vi "7HP_Pressures_to UVW.vi"(3 "Probe Number":i32) -> (1 "UVW chs":i32[](array[numeric]))   [LabVIEW 2021]
uses:
  Controls/Post_Process.ctl
  Controls/Setup.ctl
  Data plotting/MATLAB/MATLAB_Mode.ctl
  Sub_vis/Upload Data.ctl
  <vilib>/Analysis/baseanly.llb/Mean (DBL).vi
  Globals/Meas_global.vi
  Analysis/7 Hole Probe pressures to UVW/7HP_Global.vi
  Globals/Constants_global.vi
  <vilib>/Analysis/NI_AALBase.lvlib
panel:
  out "Uncorrected UVW":sgl[](array[numeric]) format="%.4f"
  out "Time to Run (s)":dbl format="%.1f"
  out "Modified Calib filename":string
  out "UVW Data?":bool
  out "RD UVW file":path
  out "RD Pressure file":path
  out "Size":i32
  out "Calib last mod":timestamp
  in  "Plot Traces":bool
  out "Array":T1(array[cluster])
  out "UVW Filepath":path
  out "UVW Sampling Rate Hz":sgl
  out "Serial number":u32
  out "Calib File":path
  out "Relative yaw (deg)":sgl
  out "Relative pitch (deg)":sgl
  out "Relative roll (deg)":sgl
  out "Calib. pitch (deg)":sgl
  out "Calib. roll (deg)":sgl
  out "Pitch (deg)":sgl
  out "Roll (deg)":sgl
  in  "Desired Freq Hz":sgl=50.0
  out "Averaging samples":i32=5
  out "Current Case":string
  out "7 Hole Probe chs":string[](array[string])
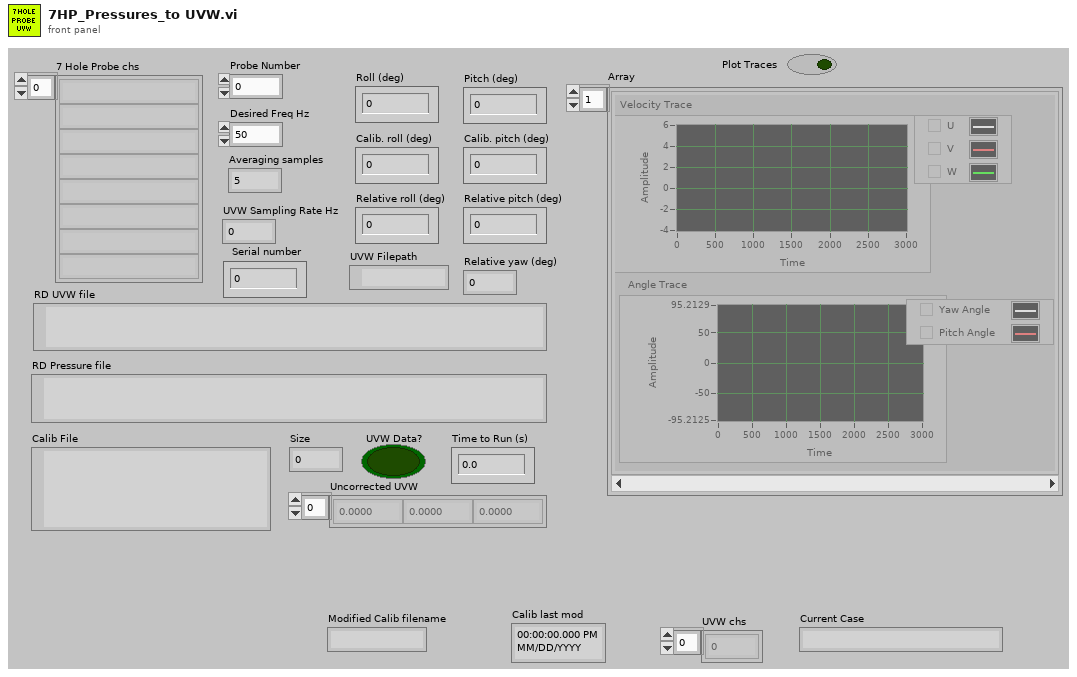
[diagram p1: front panel]
types:
  T1 = cluster{"Angle Trace":dbl[][], "Velocity Trace":sgl[][]}[]
  T2 = typedef "Post_Process.ctl" = enum16{"Take New Data", "Post Process Raw Data File"}
  T3 = typedef "Analysis_info_cluster.ctl" = cluster{"Colour":u32, "Inst type":T4, "Inst name":string, "Symbol":string, "Code name":string, "Extra Info":string, "Inst Array":T5, "Extra Titles":string[], "Extra Values":string[], "U":dbl, "u^2":dbl, "u^3":dbl, "u^4":dbl, "Skew_u":dbl, "Kurt_u":dbl, "Sd Error in Mean":dbl, "% u'/U":dbl, "X":dbl, "Y":dbl, "Z":dbl, "Timescale integral Estimate":dbl, "Sd Error in Variance":dbl, "Calib File":path, "Calib Constants":dbl[], "Output Position":bool, "Stats":enum16{"None", "Basic", "Full"}, "Av Sampling Rate":dbl, "Av No of Samples":dbl, "Total Meas Time (s)":dbl, "ADAM Ch Name":string, "Max value":dbl, "Min value":dbl, "Req Sample Rate Hz":dbl, "Sync Delay Time (s)":dbl, "Ch No":i16, "Device":string, "Use Latest Calib":bool, "Port":string, "Metadata Ch Names":string[], "Metadata Ch Values":string[], "Label":string}
  T4 = typedef "Inst_type.ctl" = enum16{"Raw voltage", "Raw with zero offsetting", "Propeller anemometer", "Pressure Transducer", "Pitot-static tube", "Hot wire", "Cross wire 1", "Cross wire 2", "Generic Linear", "Generic Polynomial", "Generic BackPoly", "Fast FID", "Thermocouple", "Cold wire", "Pulsed Wire", "LDA Vel", "LDA Tran time", "LDA Arr time", "Microphone"}
  T5 = typedef "Instrument_Array.ctl" = enum16{"PWA", "LDA", "Analogue"}
  T6 = typedef "Time_Trace_Cluster.ctl" = cluster{"Weighting":dbl[], "Voltage":dbl[], "Eng Values":dbl[]}
  T7 = typedef "Setup.ctl" = enum16{"Run Program", "Show Setup", "Save Current Setup", "Setup Front Panel"}
  T8 = enum16{"Save no data", "Save data in new files", "Save data in existing files"}
  T9 = typedef "MATLAB_Mode.ctl" = enum16{"1D Plotter", "2D Plotter", "LP Plotter", "7HP UVW"}
  T10 = typedef "Upload Data.ctl" = enum16{"Voltage Array", "Time Trace Cluster"}
  T11 = cluster{"Angle Trace":dbl[][], "Velocity Trace":sgl[][]}
  T12 = cluster{"Pressure Ch Names":string[], "Pressure Index":i32[], "Metadata Index":i32[], "Port":string}[]
  T13 = cluster{"Pressure Ch Names":string[], "Pressure Index":i32[], "Metadata Index":i32[], "Port":string}
  T14 = typedef "LVDateTimeRec.ctl" = cluster{"fractional second":dbl, "second":i32, "minute":i32, "hour":i32, "day of month":i32, "month":i32, "year":i32, "day of week":i32, "day of year":i32, "DST":i32}
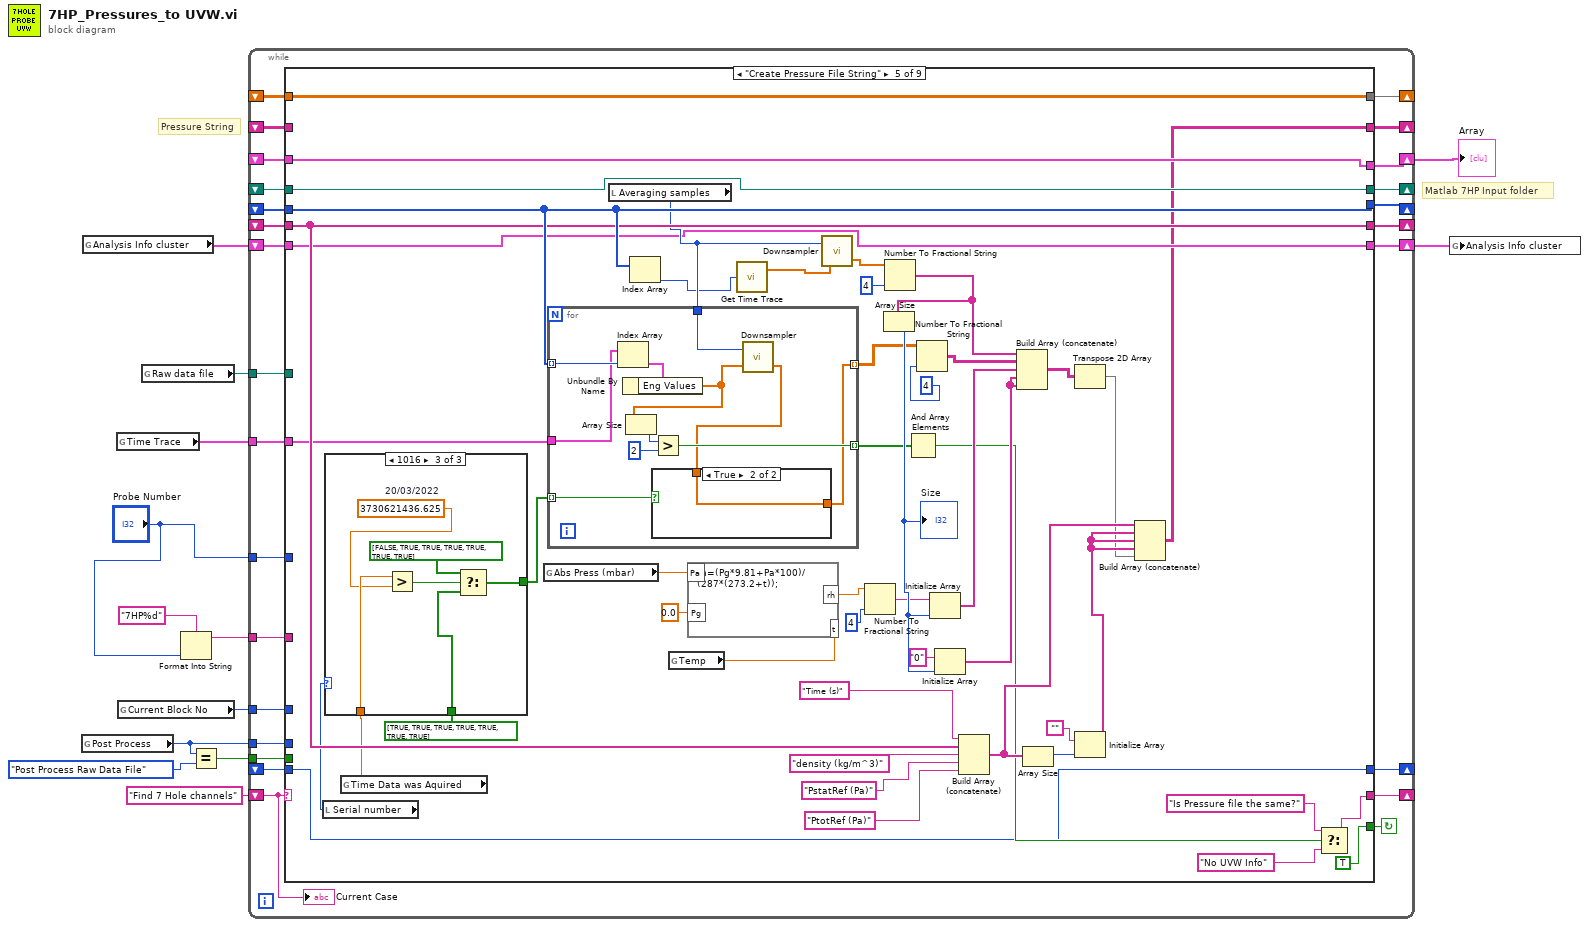
[diagram p0: block diagram]
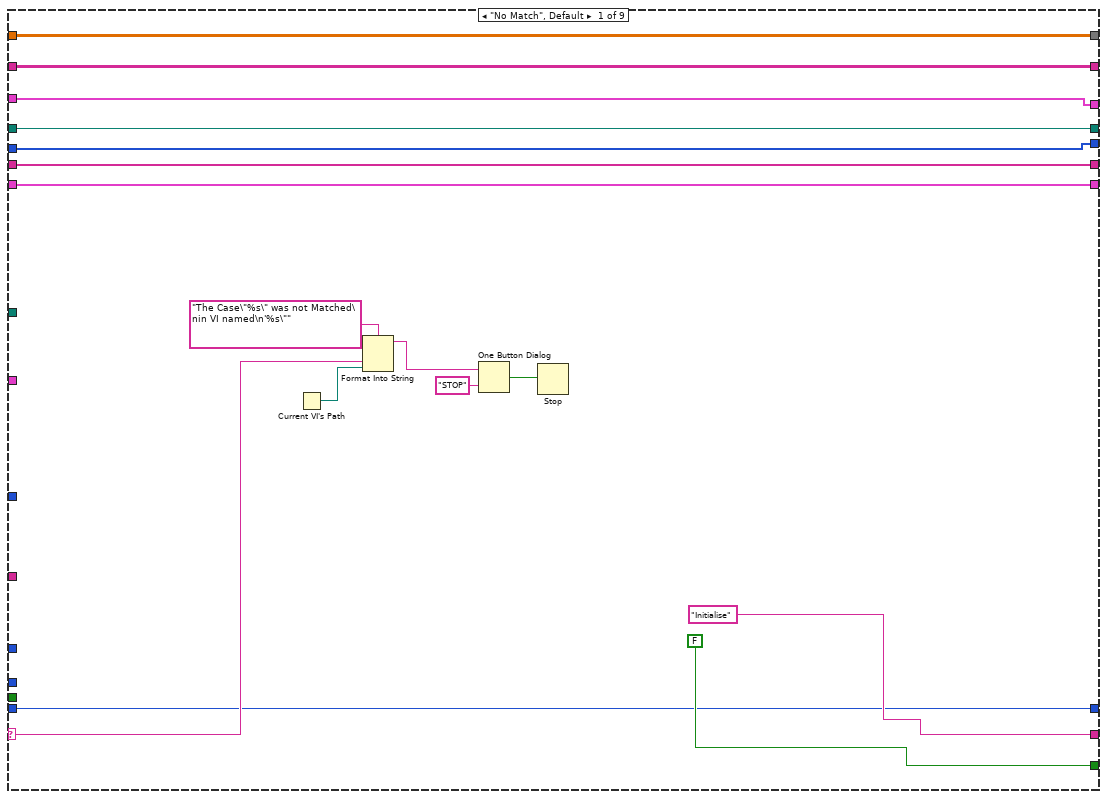
[diagram p2: hidden frame]
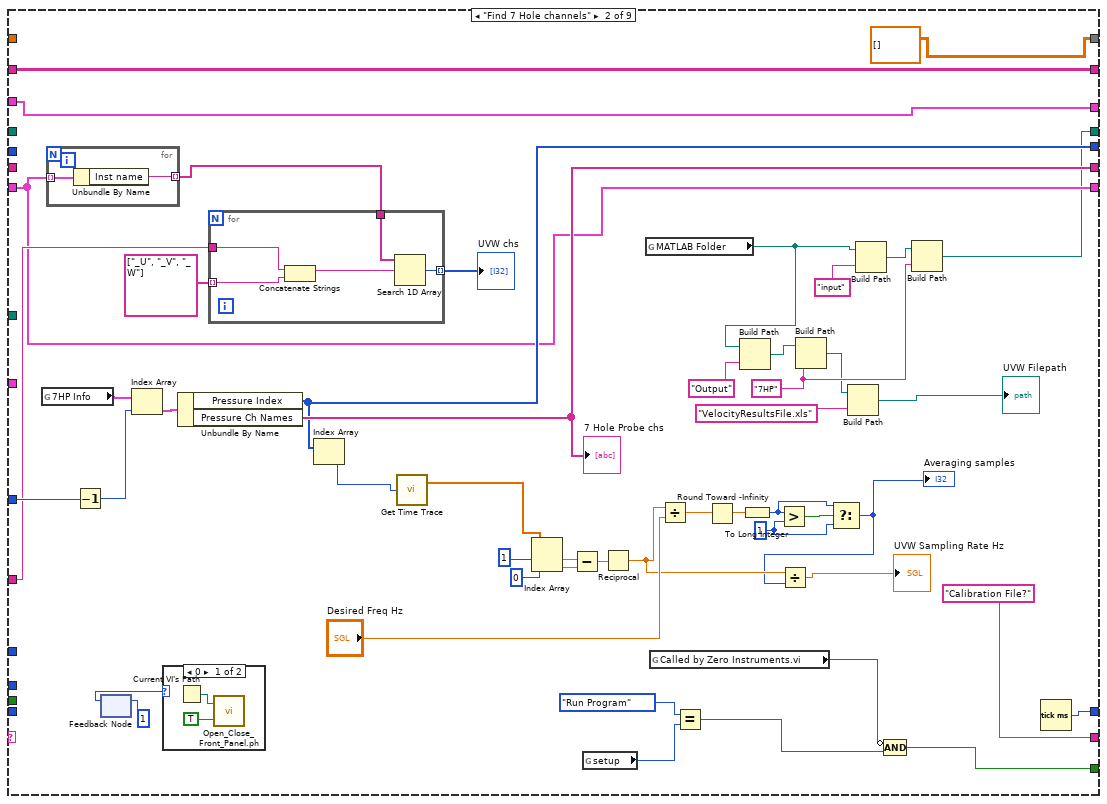
[diagram p3: hidden frame]
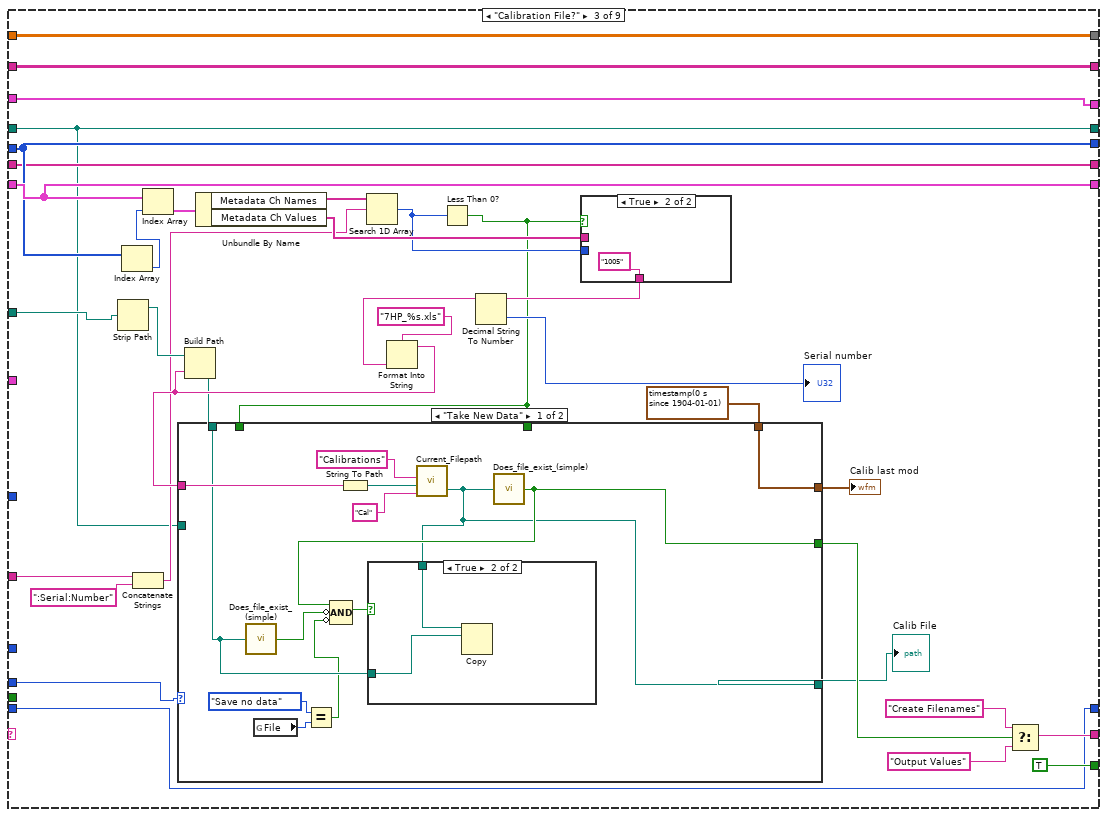
[diagram p5: hidden frame]
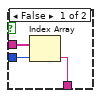
[diagram p6: hidden frame]
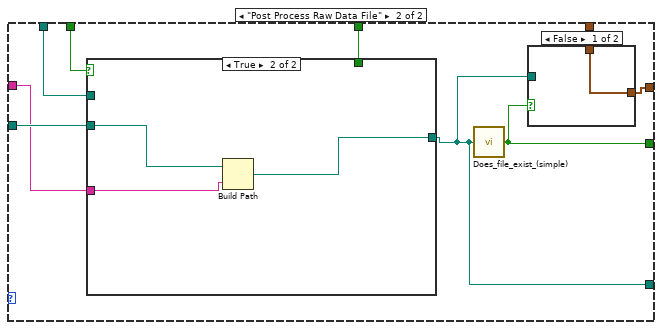
[diagram p8: hidden frame]
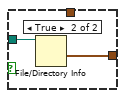
[diagram p9: hidden frame]
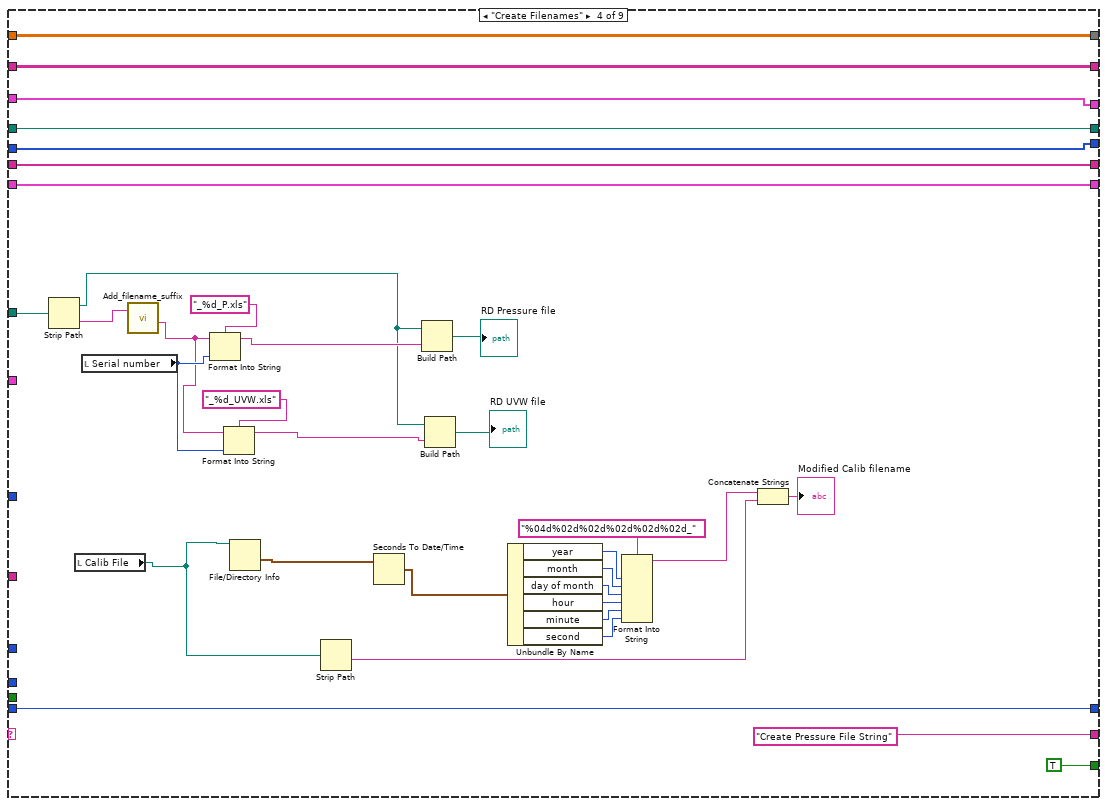
[diagram p11: hidden frame]
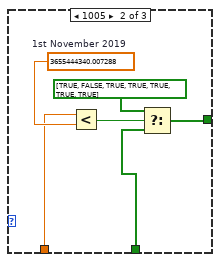
[diagram p13: hidden frame]
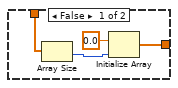
[diagram p14: hidden frame]
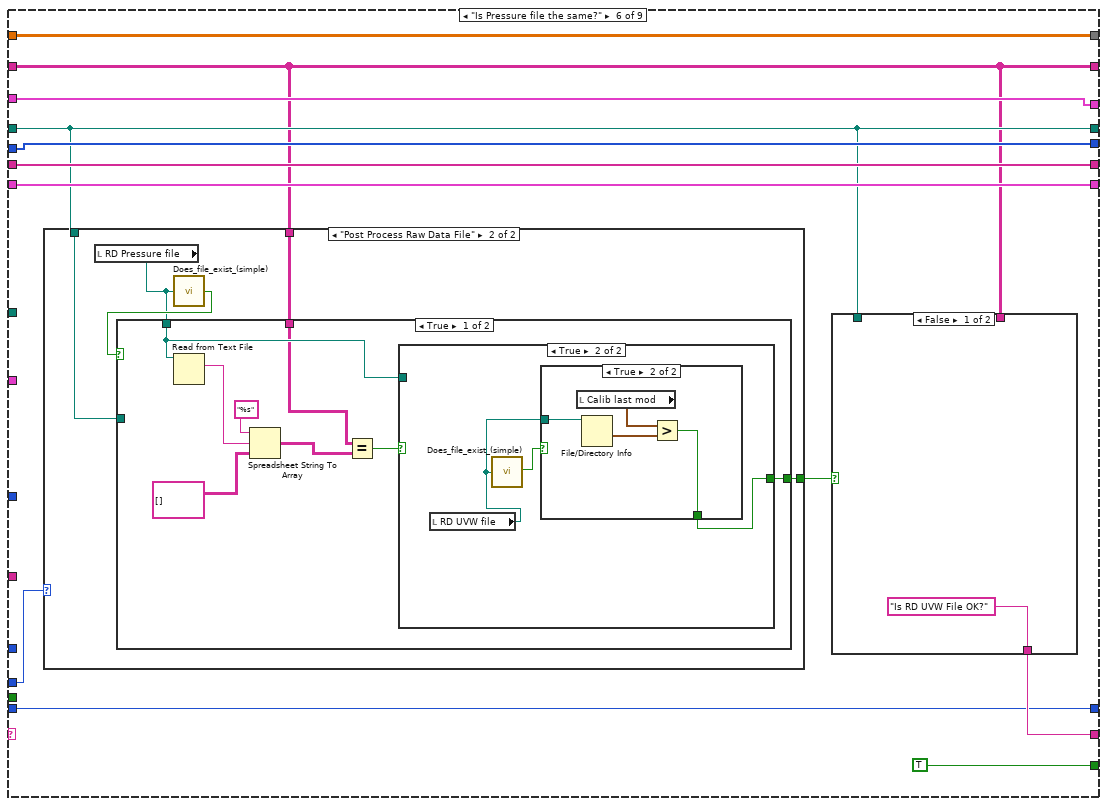
[diagram p15: hidden frame]
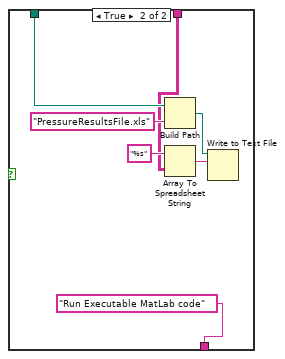
[diagram p16: hidden frame]
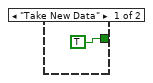
[diagram p17: hidden frame]
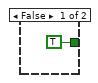
[diagram p18: hidden frame]
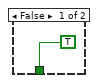
[diagram p19: hidden frame]
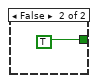
[diagram p20: hidden frame]
diagram:
  # "Matlab 7HP Input folder"
  # "Pressure String"
  n1 = global read "Meas_global.vi" "Post Process"() -> (w4:T2)
  n2 = global read "Meas_global.vi" "Analysis Info cluster"() -> (w3:T3[])
  n3 = global read "Meas_global.vi" "Time Trace"() -> (w11:T6[])
  n4 = global read "Meas_global.vi" "Current Block No"() -> (w10:i32)
  n5 = global read "Meas_global.vi" "Raw data file"() -> (w12:path)
  n6 = Format Into String(format string="7HP%d", "Probe Number") -> (resulting string=w8:string)  [unwired: 2 in, 1 out]
  n7 = Equal?(x=w4, y=Post_Process."Post Process Raw Data File" ("Post Process")) -> (x = y?=w5:bool)
  n8 = while {
    shift-left: "Find 7 Hole channels" -> [w28]
    shift-right: [w29] -> _
    tunnel: w12 -> [w38]
    shift-right: [w37] -> _
    shift-left: _ -> [w36]
    shift-right: [w35] -> _
    shift-left: _ -> [w34]
    shift-right: [w33] -> _
    shift-left: _ -> [w32]
    tunnel: w11 -> [w31]
    tunnel: w10 -> [w30]
    tunnel: "Probe Number" -> [w27]
    tunnel: w8 -> [w26]
    tunnel: w5 -> [w25]
    tunnel: w4 -> [w24]
    shift-right: [w22] -> w2
    shift-left: w3 -> [w23]
    shift-right: [w20] -> w1
    shift-left: _ -> [w21]
    shift-right: [w19] -> _
    shift-left: _ -> [w18]
    shift-right: [w17] -> _
    shift-left: _ -> [w16]
    shift-right: [w15] -> _
    shift-left: _ -> [w14]
    stop <- w39 continue-if-true
    n9 = case shown="\"Create Pressure File String\"" w28 {
      selector: w28 -> [w45 _ _ _ _ _ _ _ _]
      tunnel: [FALSE w71 TRUE TRUE TRUE TRUE TRUE TRUE FALSE] -> w39
      tunnel: ["Initialise" "Calibration File?" ("t") w131 "Create Pressure File String" ("t") w227 w294 w344 "Output Values" ("t") w445] -> w29
      tunnel: w38 -> [_ _ w136 w204 _ _ _ _ w442]
      tunnel: [w48 w93 w139 w213 w262 w303 w356 w381 w436] -> w37
      tunnel: w36 -> [w48 _ w139 w213 w262 w303 w356 w381 w443]
      tunnel: [w47 w100 w138 w212 w242 w304 w358 w382 w447] -> w35
      tunnel: w34 -> [w47 _ w138 w212 w242 w304 w358 w382 w447]
      tunnel: [w46 w80 w122 w214 w232 w296 w339 w377 w435] -> w33
      tunnel: w32 -> [w46 _ w122 w214 w232 w296 w339 w377 w434]
      tunnel: w31 -> [_ _ _ _ w236 _ _ _ w444]
      tunnel: w30 -> [_ _ _ _ _ _ _ _ _]
      tunnel: w27 -> [_ w94 _ _ _ _ _ _ w441]
      tunnel: w26 -> [_ w92 w128 _ _ _ _ _ w440]
      tunnel: w25 -> [_ _ _ _ _ _ _ _ _]
      tunnel: w24 -> [_ _ w141 _ _ w301 _ w379 _]
      tunnel: w23 -> [w44 w87 w140 w211 w233 w302 w355 w380 w438]
      tunnel: [w44 w87 w140 w211 w233 w302 w355 w380 w439] -> w22
      tunnel: w21 -> [w43 w85 w120 w215 w231 w299 w354 w376 w433]
      tunnel: [w43 w85 w120 w215 w231 w299 w354 w376 w432] -> w20
      tunnel: [w42 w84 w117 w209 w223 w295 w338 w375 w431] -> w19
      tunnel: w18 -> [w42 w84 w117 w209 _ w295 w338 w375 w431]
      tunnel: [w41 sgl[][] [] w116 w199 w224 w298 w341 w373 w430] -> w17
      tunnel: w16 -> [w41 _ w116 w199 w224 w298 w340 w372 w430]
      tunnel: [w40 w75 w115 w182 w222 w293 w337 w369 w429] -> w15
      tunnel: w14 -> [w40 _ w115 w182 w222 w293 w337 w369 w429]
      frame "No Match", Default {
        n10 = Current VI's Path() -> (path=w50:path)
        n11 = Format Into String(format string="The Case\"%s\" was not Matched\nin VI named\n'%s\"" ("Format String"), w45, w50) -> (resulting string=w53:string)  [unwired: 2 in, 1 out]
        n12 = One Button Dialog(message=w53, button name ("OK")="STOP") -> (true=w51:bool)
        n13 = Stop(stop? (T)=w51) -> ()
      }
      frame "Find 7 Hole channels" {
        w59 = 1 ("y")
        w77 = "7HP" ("name or relative path")
        n14 = global read "7HP_Global.vi" "7HP Info"() -> (w86:T12)
        n15 = for {
          tunnel: w87 -> [w108] mode=indexing
          tunnel: [w107] -> w96 mode=indexing
          n16 = Unbundle By Name(w108) -> ("Inst name"=w107:string)
        }
        n17 = Decrement(x=w94) -> (x-1=w98:i32)
        n18 = feedback-in #1(1) -> ()
        n19 = feedback #1() -> (w90:i32)  [unwired: 1 in]
        n20 = Index Array(array=w86, index=w98) -> (element=w101:T13)
        n21 = case shown="0" w90 {
          frame 0 {
            n22 = Current VI's Path() -> (path=w105:path)
            n23 = call "Open_Close_Front_Panel.ph.vi"("openWindow (T)"=TRUE ("Front Panel Window:Open"), "VI path"=w105) -> ()  [unwired: 1 in, 1 out]
          }
          frame Default {
          }
        }
        n24 = Unbundle By Name(w101) -> ("Pressure Index"=w93:i32[], "Pressure Ch Names"=w100:string[])
        "7 Hole Probe chs" <- w100
        n25 = for {
          tunnel: string[] ["_U", "_V", "_W"] ("appended array") -> [w113] mode=indexing
          tunnel: w96 -> [w112]
          tunnel: [w110] -> w95 mode=indexing
          tunnel: w92 -> [w109]
          n26 = Concatenate Strings(w109, w113) -> (w111:string)
          n27 = Search 1D Array(1D array=w112, element=w111) -> (index of element=w110:i32)  [unwired: 1 in]
        }
        "UVW chs" <- w95
        n28 = Index Array(array=w93) -> (element=w57:i32)  [unwired: 1 in]
        n29 = call "Get Time Trace.vi"("Channel Index"=w57) -> ("Time (s)"=w56:dbl[])  [unwired: 1 out]
        n30 = Index Array(array=w56, index #1=1 ("index"), index #2=0 ("index")) -> (element #1=w66:dbl, element #2=w67:dbl)
        n31 = Subtract(x=w66, y=w67) -> (x-y=w65:dbl)
        n32 = global read "Meas_global.vi" "setup"() -> (w103:T7)
        n33 = Reciprocal(x=w65) -> (1/x=w64:dbl)
        n34 = global read "Constants_global.vi" "MATLAB Folder"() -> (w74:path)
        n35 = global read "Meas_global.vi" "Called by Zero Instruments.vi"() -> (w73:bool)
        n36 = Divide(x=w64, y="Desired Freq Hz") -> (x/y=w99:dbl)
        n37 = Equal?(x=Setup."Run Program" ("setup"), y=w103) -> (x = y?=w72:bool)
        n38 = Round Toward -Infinity(1:w99) -> (0:w63:dbl)
        n39 = Build Path(base path=w74, name or relative path="Output") -> (appended path=w79:path)
        n40 = To Long Integer(number=w63) -> (32bit integer=w60:i32)
        n41 = Greater?(x=w60, y=w59) -> (0:w61:bool)
        n42 = Build Path(base path=w79, name or relative path=w77) -> (appended path=w76:path)
        n43 = Select(t=w60, s=w61, f=w59) -> (s? t:f=w58:i32)
        "Averaging samples" <- w58
        n44 = Divide(x=w64, y=w58) -> (x/y=→"UVW Sampling Rate Hz":dbl)
        n45 = Build Path(base path=w76, name or relative path="VelocityResultsFile.xls") -> (appended path=→"UVW Filepath":path)
        n46 = Build Path(base path=w74, name or relative path="input") -> (appended path=w81:path)
        n47 = Compound Arithmetic op=AND(invert w73, w72) -> (w71:bool)
        n48 = Build Path(base path=w81, name or relative path=w77) -> (appended path=w80:path)
        n49 = Tick Count (ms)() -> (millisecond timer value=w75:u32)
      }
      frame "Calibration File?" {
        n50 = Strip Path(path=w136) -> (stripped path=w137:path)  [unwired: 1 out]
        n51 = Index Array(array=w139) -> (element=w146:i32)  [unwired: 1 in]
        n52 = Concatenate Strings(w128, ":Serial:Number") -> (w127:string)
        n53 = Index Array(array=w140, index=w146) -> (element=w145:T3)
        n54 = Unbundle By Name(w145) -> ("Metadata Ch Names"=w144:string[], "Metadata Ch Values"=w143:string[])
        n55 = Search 1D Array(1D array=w144, element=w127) -> (index of element=w125:i32)  [unwired: 1 in]
        n56 = Less Than 0?(x=w125) -> (x < 0?=w123:bool)
        n57 = case shown="True" w123 {
          tunnel: w143 -> [w149 _]
          tunnel: w125 -> [w148 _]
          tunnel: [w147 "1005" ("String")] -> w124
          frame False {
            n58 = Index Array(array=w149, index=w148) -> (element=w147:string)
          }
          frame True {
          }
        }
        n59 = Format Into String(format string="7HP_%s.xls", w124) -> (resulting string=w135:string)  [unwired: 2 in, 1 out]
        n60 = Build Path(base path=w137, name or relative path=w135) -> (appended path=w134:path)
        n61 = case shown="\"Take New Data\"" w141 {
          tunnel: w135 -> [w160 w170]
          tunnel: [w159 w168] -> w132
          tunnel: w134 -> [w156 w173]
          tunnel: w123 -> [_ w174]
          tunnel: w123 -> [_ w172]
          tunnel: w122 -> [_ w171]
          tunnel: [w155 w169] -> w121
          tunnel: timestamp(0 s since 1904-01-01) ("last mod") -> [w151 w166]
          tunnel: [w151 w167] -> w118
          frame "Take New Data" {
            n62 = call "Does_file_exist_(simple).vi"("Pathname"=w156) -> ("exists?"=w158:bool)
            n63 = global read "Meas_global.vi" "File"() -> (w154:T8)
            n64 = Equal?(x=T8."Save no data" ("File"), y=w154) -> (x = y?=w152:bool)
            n65 = String To Path(string=w160) -> (path=w163:path)
            n66 = call "Current_Filepath.vi"("Short_Name"="Cal" ("Data Type"), "Filename in"=w163, "Data Type"="Calibrations") -> ("Filename Out"=w155:path)  [unwired: 1 in, 1 out]
            n67 = call "Does_file_exist_(simple).vi"("Pathname"=w155) -> ("exists?"=w159:bool)
            n68 = Compound Arithmetic op=AND(w159, invert w158, invert w152) -> (w157:bool)
            n69 = case shown="True" w157 {
              tunnel: w155 -> [_ w165]
              tunnel: w156 -> [_ w164]
              frame False {
              }
              frame True {
                n70 = Copy(10:w164, 11:w165) -> ()  [unwired: 3 in, 3 out]
              }
            }
          }
          frame "Post Process Raw Data File" {
            n71 = case shown="True" w172 {
              tunnel: w174 -> [_ _]
              tunnel: w173 -> [w178 _]
              tunnel: [w178 w179] -> w169
              tunnel: w171 -> [_ w181]
              tunnel: w170 -> [_ w180]
              frame False {
              }
              frame True {
                n72 = Build Path(base path=w181, name or relative path=w180) -> (appended path=w179:path)
              }
            }
            n73 = call "Does_file_exist_(simple).vi"("Pathname"=w169) -> ("exists?"=w168:bool)
            n74 = case shown="False" w168 {
              tunnel: w169 -> [_ w177]
              tunnel: [w175 w176] -> w167
              tunnel: w166 -> [w175 _]
              frame False {
              }
              frame True {
                n75 = File/Directory Info(path=w177) -> (last mod=w176:timestamp)  [unwired: 1 in, 6 out]
              }
            }
          }
        }
        "Calib File" <- w121
        "Calib last mod" <- w118
        n76 = Decimal String To Number(string=w124) -> (number=→"Serial number":i32)  [unwired: 2 in, 1 out]
        n77 = Select(t="Create Filenames", s=w132, f="Output Values") -> (s? t:f=w131:string)
      }
      frame "Create Filenames" {
        n78 = Strip Path(path=w204) -> (stripped path=w202:path, name=w208:string)
        n79 = local read "Calib File"() -> (w185:path)
        n80 = local read "Serial number"() -> (w207:u32)
        n81 = call "Add_filename_suffix.vi"("Filename"=w208) -> ("Base name"=w206:string)  [unwired: 1 in, 3 out]
        n82 = Format Into String(format string="_%d_P.xls", initial string=w206, w207) -> (resulting string=w203:string)  [unwired: 1 in, 1 out]
        n83 = Format Into String(format string="_%d_UVW.xls", initial string=w206, w207) -> (resulting string=w200:string)  [unwired: 1 in, 1 out]
        n84 = File/Directory Info(path=w185) -> (last mod=w188:timestamp)  [unwired: 1 in, 6 out]
        n85 = Strip Path(path=w185) -> (name=w198:string)  [unwired: 1 out]
        n86 = Seconds To Date/Time(time stamp (now)=w188) -> (date time rec=w189:T14)  [unwired: 1 in]
        n87 = Build Path(base path=w202, name or relative path=w203) -> (appended path=→"RD Pressure file":path)
        n88 = Build Path(base path=w202, name or relative path=w200) -> (appended path=→"RD UVW file":path)
        n89 = Unbundle By Name(w189) -> ("year"=w190:i32, "month"=w191:i32, "day of month"=w192:i32, "hour"=w193:i32, "minute"=w194:i32, "second"=w195:i32)
        n90 = Format Into String(format string="%04d%02d%02d%02d%02d%02d_", w190, w191, w192, w193, w194, w195) -> (resulting string=w197:string)  [unwired: 2 in, 1 out]
        n91 = Concatenate Strings(w197, w198) -> (→"Modified Calib filename":string)
      }
      frame "Create Pressure File String" {
        n92 = local read "Serial number"() -> (w221:u32)
        n93 = global read "Meas_global.vi" "Time Data was Aquired"() -> (w220:dbl)
        n94 = case shown="1016" w221 {
          tunnel: w220 -> [_ w269 w276]
          tunnel: bool[] [TRUE, TRUE, TRUE, TRUE, TRUE, TRUE, TRUE] -> [w264 w266 w273]
          tunnel: [w264 w265 w272] -> w218
          frame Default {
          }
          frame 1005 {
            w270 = 3655444340.007288  # 1st November 2019
            n95 = Less?(x=w269, y=w270) -> (x < y?=w268:bool)
            n96 = Select(t=bool[] [TRUE, FALSE, TRUE, TRUE, TRUE, TRUE, TRUE], s=w268, f=w266) -> (s? t:f=w265:bool[])
          }
          frame 1016 {
            w271 = 3730621436.625  # 20/03/2022
            n97 = Greater?(x=w276, y=w271) -> (0:w275:bool)
            n98 = Select(t=bool[] [FALSE, TRUE, TRUE, TRUE, TRUE, TRUE, TRUE], s=w275, f=w273) -> (s? t:f=w272:bool[])
          }
        }
        n99 = global read "Meas_global.vi" "Abs Press (mbar)"() -> (w260:dbl)
        n100 = local read "Averaging samples"() -> (w234:i32)
        n101 = for {
          tunnel: w262 -> [w287] mode=indexing
          tunnel: [w279] -> w230 mode=indexing
          tunnel: w236 -> [w285]
          tunnel: w234 -> [w286]
          tunnel: [w284] -> w229 mode=indexing
          tunnel: w218 -> [w277] mode=indexing
          n102 = Index Array(array=w285, index=w287) -> (element=w283:T6)
          n103 = Unbundle By Name(w283) -> ("Eng Values"=w280:dbl[])
          n104 = Array Size(array=w280) -> (size(s)=w282:i32)
          n105 = Greater?(x=w282, y=2) -> (0:w284:bool)
          n106 = call "Downsampler.vi"("Input Array"=w280, "Averaging samples"=w286) -> ("Downsampled Array"=w278:dbl[])  [unwired: 1 out]
          n107 = case shown="True" w277 {
            tunnel: [w290 w292] -> w279
            tunnel: w278 -> [w289 w292]
            frame False {
              n108 = Array Size(array=w289) -> (size(s)=w288:i32)
              n109 = Initialize Array(0.0 ("element"), w288) -> (w290:dbl[])
            }
            frame True {
            }
          }
        }
        n110 = Index Array(array=w262) -> (element=w216:i32)  [unwired: 1 in]
        n111 = global read "Meas_global.vi" "Temp"() -> (w261:dbl)
        n112 = formula code="rh=(Pg*9.81+Pa*100)/\n(287*(273.2+t));"("t"=w261, "Pg"=0.0 ("input variable"), "Pa"=w260) -> ("rh"=w245:dbl)
        n113 = call "Get Time Trace.vi"("Channel Index"=w216) -> ("Time (s)"=w217:dbl[])  [unwired: 1 out]
        n114 = call "Downsampler.vi"("Input Array"=w217, "Averaging samples"=w234) -> ("Downsampled Array"=w235:dbl[])  [unwired: 1 out]
        n115 = Number To Fractional String(number=w245, precision (6)=i16 4) -> (F-format string=w244:string)  [unwired: 2 in]
        n116 = Number To Fractional String(number=w235, precision (6)=i16 4) -> (F-format string=w249:string[])  [unwired: 2 in]
        n117 = Array Size(array=w249) -> (size(s)=w258:i32)
        "Size" <- w258
        n118 = And Array Elements(Boolean array=w229) -> (logical AND=w228:bool)
        n119 = Number To Fractional String(number=w230, precision (6)=i16 4) -> (F-format string=w247:string[][])  [unwired: 2 in]
        n120 = Initialize Array(w244, w258) -> (w256:string[])
        n121 = Initialize Array("0" ("element"), w258) -> (w255:string[])
        n122 = Build Array (concatenate)("Time (s)", w242, "density (kg/m^3)", "PstatRef (Pa)", "PtotRef (Pa)") -> (w241:string[])
        n123 = Build Array (concatenate)(w249, w247, w256, w255, w255) -> (w243:string[][])
        n124 = Array Size(array=w241) -> (size(s)=w240:i32)
        n125 = Transpose 2D Array(2D array=w243) -> (transposed array=w237:string[][])
        n126 = Initialize Array("", w240) -> (w238:string[])
        n127 = Build Array (concatenate)(w241, w238, w238, w238, w237) -> (w223:string[][])
        n128 = Select(t="Is Pressure file the same?", s=w228, f="No UVW Info") -> (s? t:f=w227:string)
      }
      frame "Is Pressure file the same?" {
        n129 = case shown="\"Post Process Raw Data File\"" w301 {
          tunnel: w296 -> [_ w317]
          tunnel: w295 -> [_ w316]
          tunnel: [TRUE w314] -> w297
          frame "Take New Data" {
          }
          frame "Post Process Raw Data File" {
            n130 = local read "RD Pressure file"() -> (w315:path)
            n131 = call "Does_file_exist_(simple).vi"("Pathname"=w315) -> ("exists?"=w318:bool)
            n132 = case shown="True" w318 {
              tunnel: w315 -> [w325 _]
              tunnel: w317 -> [_ _]
              tunnel: w316 -> [w322 _]
              tunnel: [w319 TRUE] -> w314
              frame True {
                n133 = Read from Text File(file (use dialog)=w325) -> (text=w324:string)  [unwired: 3 in, 3 out]
                n134 = Spreadsheet String To Array(format string="%s", spreadsheet string=w324, array type (2D Dbl)=string[][] []) -> (array=w321:string[][])  [unwired: 1 in]
                n135 = Equal?(x=w322, y=w321) -> (x = y?=w326:bool)
                n136 = case shown="True" w326 {
                  tunnel: w325 -> [_ _]
                  tunnel: [TRUE w328] -> w319
                  frame False {
                  }
                  frame True {
                    n137 = local read "RD UVW file"() -> (w329:path)
                    n138 = call "Does_file_exist_(simple).vi"("Pathname"=w329) -> ("exists?"=w330:bool)
                    n139 = case shown="True" w330 {
                      tunnel: w329 -> [_ w335]
                      tunnel: [TRUE w332] -> w328
                      frame False {
                      }
                      frame True {
                        n140 = local read "Calib last mod"() -> (w334:timestamp)
                        n141 = File/Directory Info(path=w335) -> (last mod=w333:timestamp)  [unwired: 1 in, 6 out]
                        n142 = Greater?(x=w334, y=w333) -> (0:w332:bool)
                      }
                    }
                  }
                }
              }
              frame False {
              }
            }
          }
        }
        n143 = case shown="False" w297 {
          tunnel: w296 -> [_ w308]
          tunnel: w295 -> [_ w307]
          tunnel: ["Is RD UVW File OK?" ("t") "Run Executable MatLab code" ("t")] -> w294
          frame False {
          }
          frame True {
            n144 = Build Path(base path=w308, name or relative path="PressureResultsFile.xls") -> (appended path=w312:path)
            n145 = Array To Spreadsheet String(array=w307, 3:"%s" ("format string")) -> (spreadsheet string=w310:string)  [unwired: 1 in]
            n146 = Write to Text File(file (use dialog)=w312, text=w310) -> ()  [unwired: 2 in, 3 out]
          }
        }
      }
      frame "Is RD UVW File OK?" {
        n147 = local read "RD UVW file"() -> (w351:path)
        n148 = Read from Text File(file (use dialog)=w351) -> (text=w353:string)  [unwired: 3 in, 3 out]
        n149 = Spreadsheet String To Array(format string="%s", spreadsheet string=w353, array type (2D Dbl)=sgl[][] []) -> (array=w352:sgl[][])  [unwired: 1 in]
        n150 = Array Subset(array=w352, index (row)=1 ("index")) -> (w342:sgl[][])  [unwired: 3 in]
        n151 = Array Size(array=w342) -> (size(s)=w347:i32[])
        n152 = local read "Size"() -> (w345:i32)
        n153 = Index Array(array=w347) -> (element=w346:i32)  [unwired: 1 in]
        n154 = Equal?(x=w345, y=w346) -> (x = y?=w343:bool)
        n155 = case shown="True" w343 {
          tunnel: ["Run Executable MatLab code" ("t") "Output Values" ("t")] -> w344
          tunnel: [w365 w367] -> w341
          tunnel: w342 -> [_ w367]
          tunnel: w340 -> [w365 _]
          tunnel: w339 -> [w360 _]
          tunnel: w338 -> [w359 _]
          frame False {
            n156 = Build Path(base path=w360, name or relative path="PressureResultsFile.xls") -> (appended path=w364:path)
            n157 = Array To Spreadsheet String(array=w359, 3:"%s" ("format string")) -> (spreadsheet string=w362:string)  [unwired: 1 in]
            n158 = Write to Text File(file (use dialog)=w364, text=w362) -> ()  [unwired: 2 in, 3 out]
          }
          frame True {
          }
        }
      }
      frame "Run Executable MatLab code" {
        # "Good data?"
        # "Error?"
        n159 = local read "Modified Calib filename"() -> (w370:string)
        n160 = local read "Calib File"() -> (w371:path)
        n161 = stacked-sequence {
          seq-local: [_ w393 _ _] -> [_ _ w400 _]
          seq-local: [_ _ w397 _] -> [_ _ _ w416]
          tunnel: w379 -> [_ _ _ w418]
          tunnel: w377 -> [w387 _ _ w417]
          tunnel: w375 -> [_ _ _ _]
          tunnel: [_ _ w399 _] -> w373
          tunnel: w372 -> [_ _ w398 _]
          tunnel: w371 -> [w386 _ _ _]
          tunnel: w370 -> [w383 w392 _ _]
          frame #0 {
            n162 = Build Path(base path=w387, name or relative path=w383) -> (appended path=w385:path)
            n163 = call "Does_file_exist_(simple).vi"("Pathname"=w385) -> ("exists?"=w384:bool)
            n164 = case shown="False" w384 {
              tunnel: w386 -> [w389 _]
              tunnel: w385 -> [w388 _]
              frame False {
                n165 = Copy(9:TRUE ("overwrite (F)"), 10:w388, 11:w389) -> ()  [unwired: 2 in, 3 out]
              }
              frame True {
              }
            }
          }
          frame #1 {
            n166 = call "Call_MATLAB_Suite.vi"("Mode"=MATLAB_Mode."7HP UVW", "Input String"=w392) -> ("error out"=w394:errorcluster)  [unwired: 1 in, 2 out]
            n167 = Unbundle By Name(w394) -> ("status"=w393:bool)
            n168 = call "EnFlo_Error_Handler.vi"("error in (no error)"=w394, "Error Type"="Run Executable MatLab Code", "Dialog Box (F)"=FALSE ("Dialog Box (T)")) -> ()  [unwired: 1 in, 2 out]
          }
          frame #2 {
            n169 = case shown="False" w400 {
              tunnel: [w402 w415] -> w399
              tunnel: w398 -> [w403 w415]
              tunnel: [w401 FALSE] -> w397
              frame False {
                n170 = local read "UVW Filepath"() -> (w411:path)
                n171 = Read from Text File(file (use dialog)=w411) -> (text=w413:string)  [unwired: 3 in, 3 out]
                n172 = Spreadsheet String To Array(format string="%s", spreadsheet string=w413, array type (2D Dbl)=sgl[][] []) -> (array=w412:sgl[][])  [unwired: 1 in]
                n173 = Array Subset(array=w412, index (row)=1 ("index")) -> (w404:sgl[][])  [unwired: 3 in]
                n174 = Array Size(array=w404) -> (size(s)=w410:i32[])
                n175 = local read "Size"() -> (w408:i32)
                n176 = Index Array(array=w410) -> (element=w409:i32)  [unwired: 1 in]
                n177 = Equal?(x=w408, y=w409) -> (x = y?=w401:bool)
                n178 = Select(t=w404, s=w401, f=w403) -> (s? t:f=w402:sgl[][])
              }
              frame True {
              }
            }
          }
          frame #3 {
            n179 = case shown="\"Post Process Raw Data File\"" w418 {
              tunnel: w416 -> [_ w420]
              tunnel: w417 -> [_ w419]
              frame "Take New Data" {
              }
              frame "Post Process Raw Data File" {
                n180 = case shown="True" w420 {
                  tunnel: w419 -> [_ w422]
                  frame False {
                  }
                  frame True {
                    n181 = local read "UVW Filepath"() -> (w427:path)
                    n182 = local read "RD UVW file"() -> (w428:path)
                    n183 = local read "RD Pressure file"() -> (w424:path)
                    n184 = Build Path(base path=w422, name or relative path="PressureResultsFile.xls") -> (appended path=w421:path)
                    n185 = Move(source path=w427, 9:TRUE ("overwrite (F)"), 10:w428) -> ()  [unwired: 2 in, 3 out]
                    n186 = Move(source path=w421, 9:TRUE ("overwrite (F)"), 10:w424) -> ()  [unwired: 2 in, 3 out]
                  }
                }
              }
            }
          }
        }
      }
      frame "Output Values" {
        # "Corr\nUVW"
        # "Orig\nUVW"
        n187 = local read "UVW chs"() -> (w437:i32[])
        n188 = stacked-sequence {
          seq-local: [_ w463 _ _ _ _] -> [_ _ w499 _ _ _]
          seq-local: [_ _ w474 _ _ _] -> [_ _ _ w560 _ _]
          seq-local: [_ _ w490 _ _ _] -> [_ _ _ _ w626 _]
          seq-local: [_ _ w471 _ _ _] -> [_ _ _ _ w627 _]
          seq-local: [w456 _ _ _ _ _] -> [_ _ w484 _ _ _]
          seq-local: [_ _ _ _ w623 _] -> [_ _ _ _ _ _]
          seq-local: [_ _ _ w564 _ _] -> [_ _ _ _ w617 _]
          seq-local: [_ _ _ w538 _ _] -> [_ _ _ _ w614 _]
          seq-local: [w454 _ _ _ _ _] -> [_ _ _ w549 _ _]
          seq-local: [w453 _ _ _ _ _] -> [_ _ _ w548 _ _]
          seq-local: [w451 _ _ _ _ _] -> [_ _ _ w546 _ _]
          seq-local: [w450 _ _ _ _ _] -> [_ _ _ w547 _ _]
          seq-local: [_ _ w476 _ _ _] -> [_ _ _ w544 _ _]
          tunnel: ["End" ("t") _ _ _ _ _] -> w445
          tunnel: w444 -> [_ w462 _ _ _ _]
          tunnel: w443 -> [_ w464 _ _ w616 _]
          tunnel: w442 -> [_ _ w488 _ _ _]
          tunnel: w441 -> [_ _ _ w559 _ _]
          tunnel: w440 -> [_ w461 _ _ w624 _]
          tunnel: [_ _ _ _ w619 _] -> w439
          tunnel: w438 -> [_ w460 _ _ w623 _]
          tunnel: w437 -> [_ _ _ w537 w620 _]
          tunnel: [_ _ _ _ w616 _] -> w436
          tunnel: [_ _ _ _ w615 _] -> w435
          tunnel: w434 -> [w448 _ _ _ w615 _]
          tunnel: w433 -> [_ _ _ w557 _ _]
          tunnel: [_ _ _ w558 _ _] -> w432
          tunnel: w430 -> [_ _ w477 w545 w612 _]
          tunnel: w429 -> [_ _ _ _ _ w656]
          frame #0 {
            n189 = local read "Modified Calib filename"() -> (w449:string)
            n190 = Build Path(base path=w448, name or relative path=w449) -> (appended path=w457:path)
            n191 = call "Get_7HP_Calib_Info.vi"("Results file"=w457) -> ("ax ay az"=w456:sgl[], "Max Min Yaw"=w455:sgl[], "Max Min Pitch"=w452:sgl[])
            n192 = Index Array(array=w455) -> (element #1=w454:sgl, element #2=w453:sgl)  [unwired: 2 in]
            n193 = Index Array(array=w452) -> (element #1=w451:sgl, element #2=w450:sgl)  [unwired: 2 in]
          }
          frame #1 {
            n194 = local read "Serial number"() -> (w459:u32)
            n195 = case shown="1000" w459 {
              tunnel: w464 -> [_ w470]
              tunnel: [sgl[] [0.0, 0.0, 1.0] ("ax ay az") w469] -> w463
              tunnel: w462 -> [_ w468]
              tunnel: w461 -> [_ w467]
              tunnel: w460 -> [_ w466]
              frame 1000 {
              }
              frame Default {
                n196 = call "7HP_Get_ax_ay_az.vi"("7HP Name"=w467, "Time Trace"=w468, "Analysis Info cluster"=w466, "Pressure Index"=w470) -> ("ax ay az"=w469:sgl[])  [unwired: 7 in]
              }
            }
          }
          frame #2 {
            # "HACK, SWAP V and W (need to fix in Matlab code\nbut will not do as this will make it incompatible with\nthe older files already post processed)"
            n197 = disable-structure shown="Enabled" {
              disable-tunnel: w488 -> [w511 _]
              disable-tunnel: [w507 sgl 0.0 ("Relative yaw (deg)")] -> w478
              frame Disabled {
                n198 = Build Array("A_Tunnel:Probe:Yaw") -> (w512:string[])
                n199 = call "Read_Chan_Value_Gen.vi"("Desired Ch Names"=w512, "Raw data file"=w511) -> ("Values"=w510:string[])  [unwired: 9 in]
                n200 = Index Array(array=w510) -> (element=w509:string)  [unwired: 1 in]
                n201 = Fract/Exp String To Number(string=w509, default (0 dbl)=sgl 0.0 ("default (0 DBL)")) -> (number=w507:sgl)  [unwired: 2 in, 1 out]
              }
              frame Enabled {
              }
            }
            "Relative yaw (deg)" <- w478
            n202 = Array Subset(array=w477, index (col)=1 ("index"), length (col)=3 ("length")) -> (w486:sgl[][])  [unwired: 2 in]
            n203 = for {
              tunnel: w486 -> [w520] mode=indexing
              tunnel: [w518] -> w476 mode=indexing
              n204 = Index Array(array=w520) -> (element #1=w519:sgl, element #2=w516:sgl, element #3=w517:sgl)  [unwired: 3 in]
              n205 = Negate(x=w516) -> (-x=w515:sgl)
              n206 = Build Array(w519, w517, w515) -> (w518:sgl[])
            }
            n207 = Index Array(array=w484) -> (element #1=w483:sgl, element #2=w482:sgl, element #3=w481:sgl)  [unwired: 3 in]
            n208 = Index Array(array=w499) -> (element #1=w498:sgl, element #2=w497:sgl, element #3=w496:sgl)  [unwired: 3 in]
            n209 = Negate(x=w478) -> (-x=w485:sgl)
            n210 = call "Probe orientation info.vi"("az"=w496, "ax_cal"=w483, "ay"=w497, "ax"=w498, "az_cal"=w481, "ay_cal"=w482) -> ("Relative roll (deg)"=w480:sgl, "Calib. pitch (deg)"=w491:sgl, "Calib. roll (deg)"=w487:sgl, "Pitch (deg)"=w492:sgl, "Relative pitch (deg)"=w479:sgl, "Roll (deg)"=w493:sgl)
            "Roll (deg)" <- w493
            "Pitch (deg)" <- w492
            "Calib. roll (deg)" <- w487
            "Calib. pitch (deg)" <- w491
            "Relative roll (deg)" <- w480
            "Relative pitch (deg)" <- w479
            n211 = call "UVW orientation correction.vi"("(U, V, W) array in"=w476, "Relative yaw (deg)"=w485, "Relative pitch (deg)"=w479, "Relative roll (deg)"=w480) -> ("(U, V, W) array out"=w474:sgl[][])  [unwired: 5 in]
            n212 = for {
              N: 3 -> [_]
              tunnel: w474 -> [w506]
              tunnel: [w501] -> w472 mode=indexing
              i -> [w505]
              n213 = Index Array(array=w506, index (col)=w505) -> (element=w504:sgl[])  [unwired: 1 in]
              n214 = Add Array Elements(numeric array=w504) -> (sum=w503:sgl)
              n215 = Array Size(array=w504) -> (size(s)=w502:i32)
              n216 = To Single Precision Float(number=w502) -> (single precision float=w500:sgl)
              n217 = Divide(x=w503, y=w500) -> (x/y=w501:sgl)
            }
            n218 = for {
              N: 3 -> [_]
              tunnel: w476 -> [w527]
              tunnel: [w522] -> w473 mode=indexing
              i -> [w526]
              n219 = Index Array(array=w527, index (col)=w526) -> (element=w525:sgl[])  [unwired: 1 in]
              n220 = Add Array Elements(numeric array=w525) -> (sum=w524:sgl)
              n221 = Array Size(array=w525) -> (size(s)=w523:i32)
              n222 = To Single Precision Float(number=w523) -> (single precision float=w521:sgl)
              n223 = Divide(x=w524, y=w521) -> (x/y=w522:sgl)
            }
            n224 = Build Array(w493, w492, w487, w491, w480, w479, w478) -> (w490:sgl[])
            n225 = Build Array (concatenate)(w473, w472) -> (w471:sgl[])
            "Uncorrected UVW" <- w471
          }
          frame #3 {
            n226 = Transpose 2D Array(2D array=w560) -> (transposed array=w536:sgl[][])
            n227 = Index Array(array=w545, index (col)=0 ("disabled index (col)")) -> (element=w534:sgl[])  [unwired: 1 in]
            n228 = Array Size(array=w560) -> (size(s)=w567:i32[])
            n229 = Divide(x=180.0, y=3.141592653589793) -> (x/y=w563:dbl)
            n230 = Index Array(array=w567) -> (element #1=w554:i32, element #2=w530:i32)  [unwired: 2 in]
            n231 = Index Array(array=w534) -> (element #1=w532:sgl, element #2=w533:sgl)  [unwired: 2 in]
            n232 = for {
              tunnel: w544 -> [w605] mode=indexing
              tunnel: w563 -> [w597]
              tunnel: [w594] -> w543 mode=indexing
              tunnel: [w591] -> w542 mode=indexing
              shift-right: [w595] -> w555
              shift-left: 0 -> [w596]
              tunnel: w549 -> [w593]
              tunnel: w548 -> [w592]
              tunnel: w547 -> [w590]
              tunnel: w546 -> [w589]
              n233 = Index Array(array=w605) -> (element #1=w599:sgl, element #2=w604:sgl, element #3=w598:sgl)  [unwired: 3 in]
              n234 = Divide(x=w604, y=w599) -> (x/y=w603:sgl)
              n235 = Divide(x=w598, y=w599) -> (x/y=w600:sgl)
              n236 = Inverse Tangent(1:w603) -> (0:w602:sgl)
              n237 = Inverse Tangent(1:w600) -> (0:w601:sgl)
              n238 = Multiply(x=w602, y=w597) -> (x*y=w594:dbl)
              n239 = Multiply(x=w601, y=w597) -> (x*y=w591:dbl)
              n240 = In Range and Coerce(upper limit=w593, x=w594, lower limit=w592) -> (In Range?=w588:bool)  [unwired: 1 out]
              n241 = In Range and Coerce(upper limit=w589, x=w591, lower limit=w590) -> (In Range?=w587:bool)  [unwired: 1 out]
              n242 = And(x=w588, y=w587) -> (x .and. y?=w586:bool)
              n243 = case shown="True" w586 {
                tunnel: w596 -> [w607 w608]
                tunnel: [w606 w608] -> w595
                frame False {
                  n244 = Increment(x=w607) -> (x+1=w606:i32)
                }
                frame True {
                }
              }
            }
            n245 = Subtract(x=w533, y=w532) -> (x-y=w531:sgl)
            n246 = Reciprocal(x=w531) -> (1/x=w529:sgl)
            n247 = Initialize Array(w529, w530) -> (w528:sgl[])
            n248 = Array Max & Min(array=w534) -> (max value=w566:sgl, min value=w565:sgl)  [unwired: 2 out]
            n249 = Subtract(x=w566, y=w565) -> (x-y=w564:sgl)
            n250 = call "Load_Analogue_Data_2_Time_traces.vi"("Sampling Rate (Hz)"=w528, "Mode"=Upload_Data."Voltage Array", "Index"=w537, "Voltage Array"=w536) -> ()  [unwired: 3 in]
            n251 = case shown="True" "Plot Traces" {
              tunnel: w543 -> [_ w580]
              tunnel: w542 -> [_ w579]
              tunnel: w536 -> [_ w577]
              tunnel: w559 -> [_ w576]
              tunnel: [w569 w574] -> w558
              tunnel: w557 -> [_ w573]
              tunnel: T11 {"Angle Trace"=[], "Velocity Trace"=[]} ("Cluster") -> [w571 w572]
              frame False {
                n252 = Initialize Array(w571, 0 ("dimension size")) -> (w569:T1)
              }
              frame True {
                n253 = Build Array(w580, w579) -> (w578:dbl[][])
                n254 = Bundle By Name(cluster=w572, "Angle Trace"=w578, "Velocity Trace"=w577) -> (w575:T11)
                n255 = case shown="Default" w576 {
                  tunnel: w575 -> [w583 w585]
                  tunnel: [w582 w584] -> w574
                  tunnel: w573 -> [w581 _]
                  frame Default {
                    n256 = Build Array (concatenate)(w581, w583) -> (w582:T1)
                  }
                  frame 1 {
                    n257 = Build Array(w585) -> (w584:T1)
                  }
                }
              }
            }
            n258 = Divide(x=w555, y=w554) -> (x/y=w553:dbl)
            n259 = Multiply(x=w553, y=100.0) -> (x*y=w541:dbl)
            n260 = call-poly <vilib>:"Mean.vi"("X"=w543) -> ("mean"=w540:dbl)  [unwired: 1 out]
            n261 = call-poly <vilib>:"Mean.vi"("X"=w542) -> ("mean"=w539:dbl)  [unwired: 1 out]
            n262 = Build Array(w541, w540, w539) -> (w538:dbl[])
          }
          frame #4 {
            n263 = local read "UVW Sampling Rate Hz"() -> (w618:sgl)
            n264 = Build Array (concatenate)(w626, w627, w618, w614) -> (w625:dbl[])
            n265 = Array Size(array=w612) -> (size(s)=w611:i32[])
            n266 = Index Array(array=w611) -> (element=w610:i32)  [unwired: 1 in]
            n267 = for {
              tunnel: w624 -> [w651]
              tunnel: string[] [":Roll:(deg)", ":Pitch:(deg)", ":Calib Roll:(deg)", ":Calib Pitch:(deg)", ":Relative Roll:(deg)", ":Relative Pitch:(deg)", ":Relative Yaw:(deg)", ":Uncorrected:U", ":Uncorrected:V", ":Uncorrected:W", ":U:m/s", ":V:m/s", ":W:m/s", ":UVW Data Rate:(Hz)", ":Outside:Calibration %", ":Uncorrected:Yaw From Flow", ":Uncorrected:Pitch From Flow"] -> [w650] mode=indexing
              tunnel: w625 -> [w648] mode=indexing
              tunnel: [w647] -> w629 mode=indexing
              tunnel: [w646] -> w628 mode=indexing
              n268 = Concatenate Strings(w651, w650) -> (w647:string)
              n269 = Number To Fractional String(number=w648, precision (6)=i16 4) -> (F-format string=w646:string)  [unwired: 2 in]
            }
            n270 = Greater Than 0?(x=w610) -> (x > 0?=w609:bool)
            "UVW Data?" <- w609
            n271 = Index Array(array=w616) -> (element=w622:i32)  [unwired: 1 in]
            n272 = in-place {
              in-place-border: w629 -> [w644]
              in-place-border: w628 -> [w643]
              n273 = in-place-array #2(w623, w622) -> (w642:T3)
              n274 = call "Update Metadata channels.vi"("Metadata Values"=w643, "Metadata Names"=w644, "Analysis info Cluster in"=w642) -> ("Analysis info Cluster out"=w645:T3)
              n275 = in-place-array #2(w645) -> (w621:T3[])  [unwired: 1 out]
            }
            n276 = case shown="True" w609 {
              tunnel: [enum16{"None", "Basic", "Full"}."None" ("Stats") enum16{"None", "Basic", "Full"}."Full" ("Stats")] -> w613
              frame False {
              }
              frame True {
              }
            }
            n277 = for {
              shift-right: [w635] -> w619
              shift-left: w621 -> [w636]
              tunnel: w620 -> [w637] mode=indexing
              tunnel: w617 -> [w634]
              tunnel: w613 -> [w633]
              n278 = in-place {
                in-place-border: w634 -> [w639]
                in-place-border: w633 -> [w638]
                n279 = in-place-array #3(w636, w637) -> (w641:T3)
                n280 = Bundle By Name(cluster=w641, "Total Meas Time (s)"=w639, "Stats"=w638) -> (w640:T3)
                n281 = in-place-array #3(w640) -> (w635:T3[])  [unwired: 1 out]
              }
            }
          }
          frame #5 {
            n282 = Tick Count (ms)() -> (millisecond timer value=w655:u32)
            n283 = Subtract(x=w655, y=w656) -> (x-y=w653:u32)
            n284 = Divide(x=w653, y=u32 1000) -> (x/y=→"Time to Run (s)":dbl)
          }
        }
      }
    }
    "Current Case" <- w28
  }
  "Array" <- w1
  n285 = global write "Meas_global.vi" "Analysis Info cluster"(w2) -> ()
